vi "Example.vi"() -> ()   [LabVIEW 2014, in "Sixpack - Driver.lvlib"]
uses:
  Sixpack - Driver.lvlib
panel:
  out "error out":errorcluster
  out "time to poll":u32 caption="ms"
  in  "TargetPosition":i32
  out "CurrentPosition":i32
  in  "MotNr(0..5)":u8
  in  "UnitAddress(0)":u16
  in  "Stop":bool
  in  "BaudRate (19200)":enum32{"9600", "19200", "38400", "57600"}(ring)=enum."19200"
  in  "COM Port (COM1)":T1(ring)
  out "handle":i32
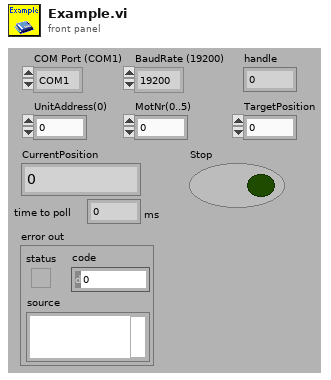
[diagram p1: front panel]
types:
  T1 = enum32{"COM1", "COM2", "COM3", "COM4", "COM5", "COM6", "COM7", "COM8", "COM9"}
  T2 = typedef "Sixpack - Driver.lvlib/Activity.ctl" = enum16{"Inactive", "Ramp", "PI-Controller", "Rotation", "ReferenceSearch", "Reference Search", "MechanicalReference"}
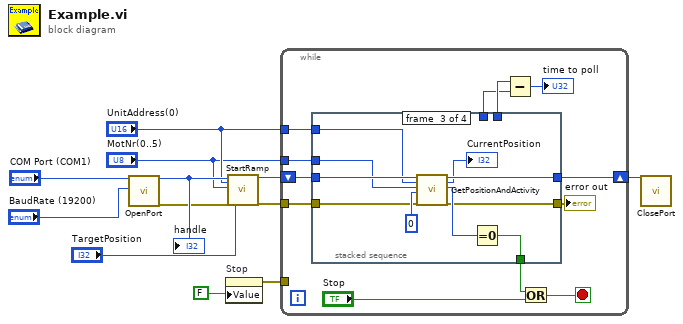
[diagram p0: block diagram]
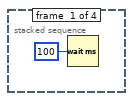
[diagram p2: hidden frame]
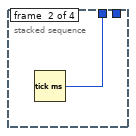
[diagram p3: hidden frame]
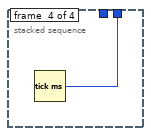
[diagram p4: hidden frame]
diagram:
  n1 = call "OpenPort.vi"("COM Port (COM1)"="COM Port (COM1)", "BaudRate (19200)"="BaudRate (19200)") -> ("handle"=w10:i32, "error out"=w2:errorcluster)  [unwired: 16 in]
  "handle" <- w10
  n2 = property on="Stop" class="Bool (strict)"("Value"=FALSE ("Stop")) -> (error out=w5:errorcluster)  [unwired: 2 in, 1 out]
  n3 = call "StartRamp.vi"("handle in"=w10, "UnitAddress(0)"="UnitAddress(0)", "MotNr(0)"="MotNr(0..5)", "error in"=w2, "TargetPosition(0)"="TargetPosition") -> ("handle out"=w9:i32, "error out"=w1:errorcluster)  [unwired: 13 in]
  n4 = while {
    shift-right: [w23] -> w8
    shift-left: w9 -> [w24]
    tunnel: "UnitAddress(0)" -> [w22]
    tunnel: "MotNr(0..5)" -> [w21]
    tunnel: w5 -> [_]
    tunnel: w1 -> [w14]
    stop <- w17 stop-if-true
    n5 = stacked-sequence {
      tunnel: w24 -> [_ _ w36 _]
      tunnel: [_ _ w35 _] -> w23
      tunnel: w22 -> [_ _ w32 _]
      tunnel: w21 -> [_ _ w31 _]
      tunnel: [_ w26 _ _] -> w19
      tunnel: [_ _ _ w37] -> w20
      tunnel: [_ _ w29 _] -> w15
      tunnel: w14 -> [_ _ w28 _]
      tunnel: [_ _ w27 _] -> w13
      frame #0 {
        n6 = Wait (ms)(milliseconds to wait=u32 100) -> ()  [unwired: 1 out]
      }
      frame #1 {
        n7 = Tick Count (ms)() -> (millisecond timer value=w26:u32)
      }
      frame #2 {
        n8 = call "GetPositionAndActivity.vi"("handle in"=w36, "UnitAddress(0)"=w32, "MotNr(0)"=w31, "ResponseAddress(0)"=u8 0, "error in"=w28) -> ("handle out"=w35:i32, "CurrentPosition"=→"CurrentPosition":i32, "CurrentActivity"=w30:T2, "error out"=w27:errorcluster)  [unwired: 10 in, 1 out]
        n9 = Equal To 0?(x=w30) -> (x = 0?=w29:bool)
      }
      frame #3 {
        n10 = Tick Count (ms)() -> (millisecond timer value=w37:u32)
      }
    }
    "error out" <- w13
    n11 = Subtract(x=w20, y=w19) -> (x-y=→"time to poll":u32)
    n12 = Or(x=w15, y="Stop") -> (x .or. y?=w17:bool)
  }
  n13 = call "ClosePort.vi"("handle"=w8) -> ()  [unwired: 19 in]
